vi "Splash Screen.vi"() -> (0 "Boolean":bool=TRUE)   [LabVIEW 2017]
panel:
  out "Horizontal Progress Bar":u8(slide) scale=0.0..100.0
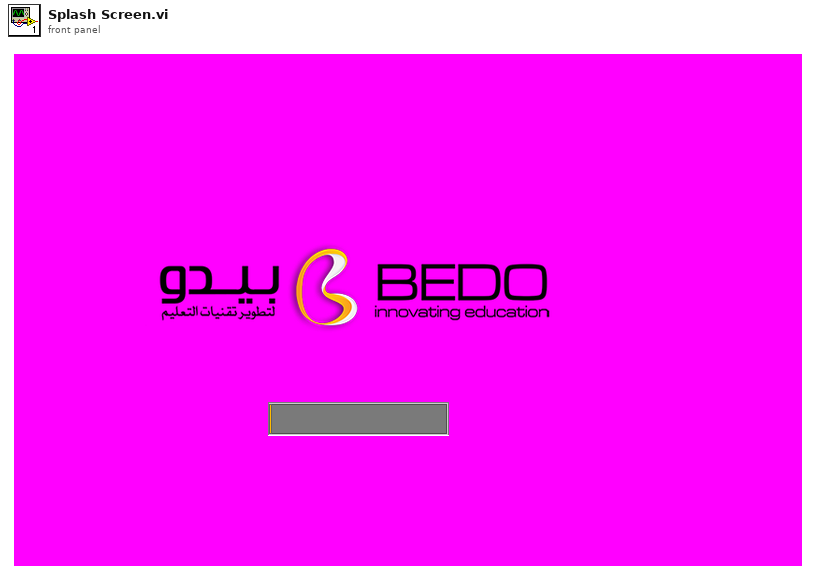
[diagram p1: front panel]
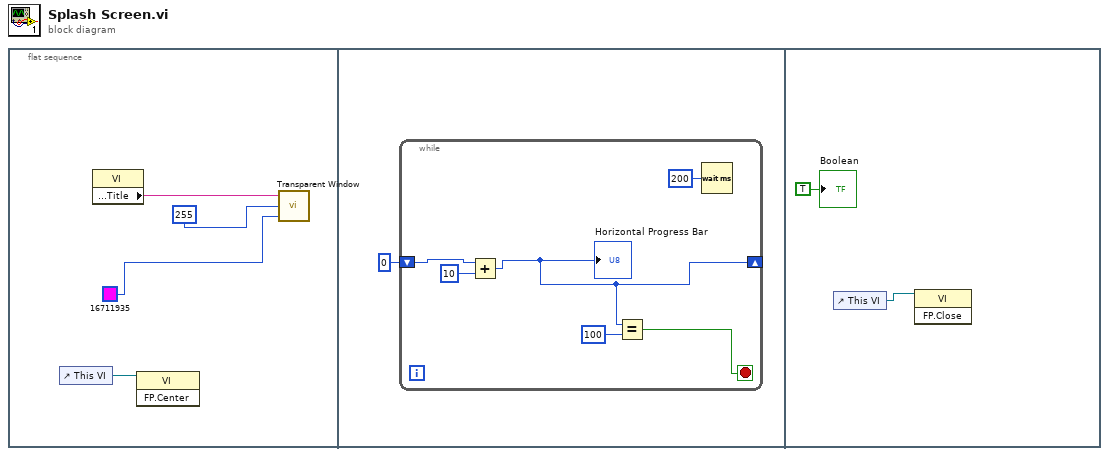
[diagram p0: block diagram]
diagram:
  n1 = flat-sequence {
    frame #0 {
      n2 = control-ref of="This VI"() -> (w1:refnum<vi>)
      n3 = property class="VI"() -> ("Front Panel.Title"=w4:string)  [unwired: 2 in, 2 out]
      n4 = invoke class="VI" method="FP.Center"(reference=w1) -> ()  [unwired: 2 in, 3 out]
      n5 = call "Transparent Window.vi"("crkey"=u32 16711935 ("Color Box 2"), "Slide"=u8 255, "window name (\"\")"=w4) -> ()  [unwired: 1 in]
    }
    frame #1 {
      n6 = while {
        shift-right: [w8] -> _
        shift-left: u8 0 -> [w9]
        stop <- w6 stop-if-true
        n7 = Add(x=w9, y=u8 10) -> (x+y=w8:u8)
        "Horizontal Progress Bar" <- w8
        n8 = Equal?(x=w8, y=u8 100) -> (x = y?=w6:bool)
        n9 = Wait (ms)(milliseconds to wait=u32 200) -> ()  [unwired: 1 out]
      }
    }
    frame #2 {
      n10 = control-ref of="This VI"() -> (w12:refnum<vi>)
      n11 = invoke class="VI" method="FP.Close"(reference=w12) -> ()  [unwired: 2 in, 3 out]
      "Boolean" <- TRUE
    }
  }
